vi "Read FFT Measurement Peak Search Result.vi"(8 "error in (no error)":errorcluster, 9 "Result Type (Current)":i32(ring) items=["Current", "Average"], 10 "Instance (1)":i32=1, 11 "VISA resource name":refnum<visa-resource-name>) -> (0 "error out":errorcluster, 1 "Power":dbl[](array[numeric]) format="%^.3e", 2 "Reliability":i32, 3 "VISA resource name out":refnum<visa-resource-name>, 4 "Frequency":dbl[](array[numeric]) format="%#.9p")   [LabVIEW 2015, in "Rohde&Schwarz CMXP GPRF.lvlib"]
doc: "Starts a new single shot measurement and returns the results of the peak search.\n\nAttributes:\nRSCMXPGPRF_ATTR_READ_FFT_MEASUREMENT_PEAK_SEARCH_RESULT_CURRENT\nRSCMXPGPRF_ATTR_READ_FFT_MEASUREMENT_PEAK_SEARCH_RESULT_AVERAGE\n\nRemote-control commands:\nREAD:GPRF:MEAS<i>:FFTSanalyzer:PEAKs:CURRent?\nREAD:GPRF:MEAS<i>:FFTSanalyzer:PEAKs:AVERage?"
uses:
  <instrlib>/Rohde&Schwarz CMXP GPRF/Rohde&Schwarz CMXP GPRF.lvlib
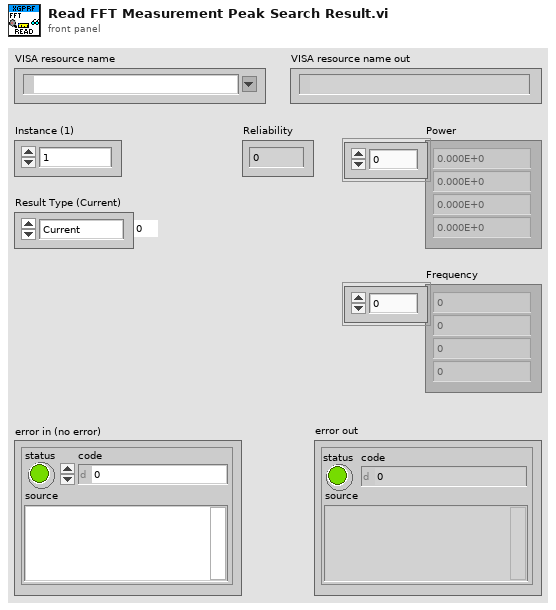
[diagram p1: front panel]
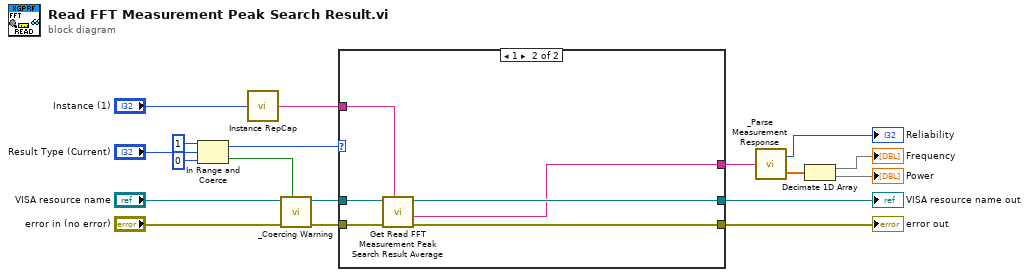
[diagram p0: block diagram]
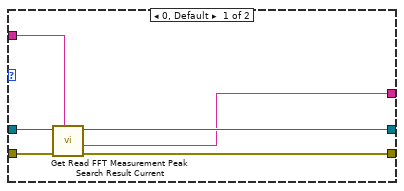
[diagram p2: hidden frame]
diagram:
  n1 = In Range and Coerce(upper limit=1, x="Result Type (Current)", lower limit=0) -> (coerced(x)=w10:i32, In Range?=w5:bool)
  n2 = call <instrlib>:"Instance RepCap.vi"("instance  in"="Instance (1)") -> ("instance out"=w11:string)
  n3 = call <instrlib>:"_Coercing Warning.vi"("In Range?"=w5, "error in (no error)"="error in (no error)", "VISA resource name"="VISA resource name") -> ("error out"=w9:errorcluster, "VISA resource name out"=w8:refnum<visa-resource-name>)  [unwired: 7 in]
  n4 = case shown="1" w10 {
    tunnel: w11 -> [w20 w26]
    tunnel: w9 -> [w24 w30]
    tunnel: w8 -> [w23 w29]
    tunnel: [w22 w28] -> w7
    tunnel: [w21 w27] -> w6
    tunnel: [w19 w25] -> w3
    frame 0, Default {
      n5 = call "Get Read FFT Measurement Peak Search Result Current"("Repeated Capabilities"=w20, "error in (no error)"=w24, "instrument handle"=w23) -> ("error out"=w22:errorcluster, "Read FFT Measurement Peak Search Result Current"=w19:string, "instrument handle out"=w21:refnum<visa-resource-name>)  [unwired: 6 in]
    }
    frame 1 {
      n6 = call "Get Read FFT Measurement Peak Search Result Average"("Repeated Capabilities"=w26, "error in (no error)"=w30, "instrument handle"=w29) -> ("error out"=w28:errorcluster, "Read FFT Measurement Peak Search Result Average"=w25:string, "instrument handle out"=w27:refnum<visa-resource-name>)  [unwired: 6 in]
    }
  }
  "error out" <- w7
  "VISA resource name out" <- w6
  n7 = call <instrlib>:"_Parse Measurement Response.vi"("String In"=w3) -> ("Reliability"=→"Reliability":i32, "Data"=w1:dbl[])
  n8 = Decimate 1D Array(w1) -> (→"Frequency":dbl[], →"Power":dbl[])
